vi "Initialize Movement Task.vi"(0 "NI Force Task in":refnum<class "NI Force Task.lvclass">, 1 "Pot Calibration Cluster":cluster{"Left":dbl, "Right":dbl}, 2 "TDMS File":refnum<k34>, 3 "EMG info":cluster{"Collect EMG?":bool, "EMG Rate":u16}, 4 "DAQ  Channels In":T1={"Force Transducer: Left"="Dev1/ai6", "Force Transducer: Right "="Dev1/ai8", "EMG: Left"="", "EMG: Right"="", "Potentiometer: Left"="", "Potentiometer: Right"=""}, 5 "error in (no error)":errorcluster, 7 "Task Info In":T2={"Number of Trials"=1, "Sampling Rate (Hz)"=200, "Trial Duration (s)"=10, "Adjusted MVC (N)"=5.0, "R Phase"=0, "L Phase"=0, "L Pattern"=1, "R Pattern"=1, "Time Between Trials (s)"=5, "Lissajous Speed"=200} {"Lissajous Speed" min=1 max=200; "Time Between Trials (s)" min=1 step=1; "R Pattern" min=1 max=20 step=1; "L Pattern" min=1 max=20 step=1; "L Phase" max=360 step=1; "R Phase" max=360 step=1; "Adjusted MVC (N)" min=1.0 step=1.0; "Trial Duration (s)" min=1 step=1; "Sampling Rate (Hz)" min=1 step=1; "Number of Trials" min=1 step=1}, 9 "Scanning?":bool=TRUE) -> (14 "NI Force Task out":refnum<class "NI Force Task.lvclass">, 19 "error out":errorcluster)   [LabVIEW 2020, in "NI Force Task.lvlib" / "NI Force Task.lvclass"]
uses:
  NI Force Task.lvclass
  C:/Program Files/National Instruments/LabVIEW 2020/vi.lib/ActorFramework/Actor/Actor.lvclass
  Task info df.ctl
  <vilib>/ActorFramework/Message Enqueuer/Message Priority.ctl
  <vilib>/ActorFramework/Actor/Actor.lvclass/Actor.ctl
  <vilib>/ActorFramework/Message Enqueuer/Message Enqueuer.lvclass/Message Enqueuer.ctl
  NI Force Task.lvclass/NI Force Task.ctl
  NI Force Task Messages/Update Template Graph Msg/Update Template Graph Msg.lvclass/Update Template Graph Msg.ctl
  <vilib>/ActorFramework/Message Enqueuer/Init from Existing Queue.vi
  <vilib>/ActorFramework/Message Enqueuer/Enqueue.vi
  NI Force Task Messages/Update Template Graph Msg/Update Template Graph Msg.lvclass
  C:/Program Files/National Instruments/LabVIEW 2020/vi.lib/ActorFramework/Message/Message.lvclass
  <vilib>/ActorFramework/Message Priority Queue/Priority Enqueue.vi
  <vilib>/DAQmx/create/channels.llb/DAQmx Create Channel (AI-Voltage-Basic).vi
  <vilib>/DAQmx/configure/timing.llb/DAQmx Timing (Sample Clock).vi
  <vilib>/ActorFramework/Message Enqueuer/Message Enqueuer.lvclass
  <vilib>/ActorFramework/Actor/Actor.lvclass
panel:
  out "error out 2":errorcluster
  # "Left Arm"
  # "Right Arm"
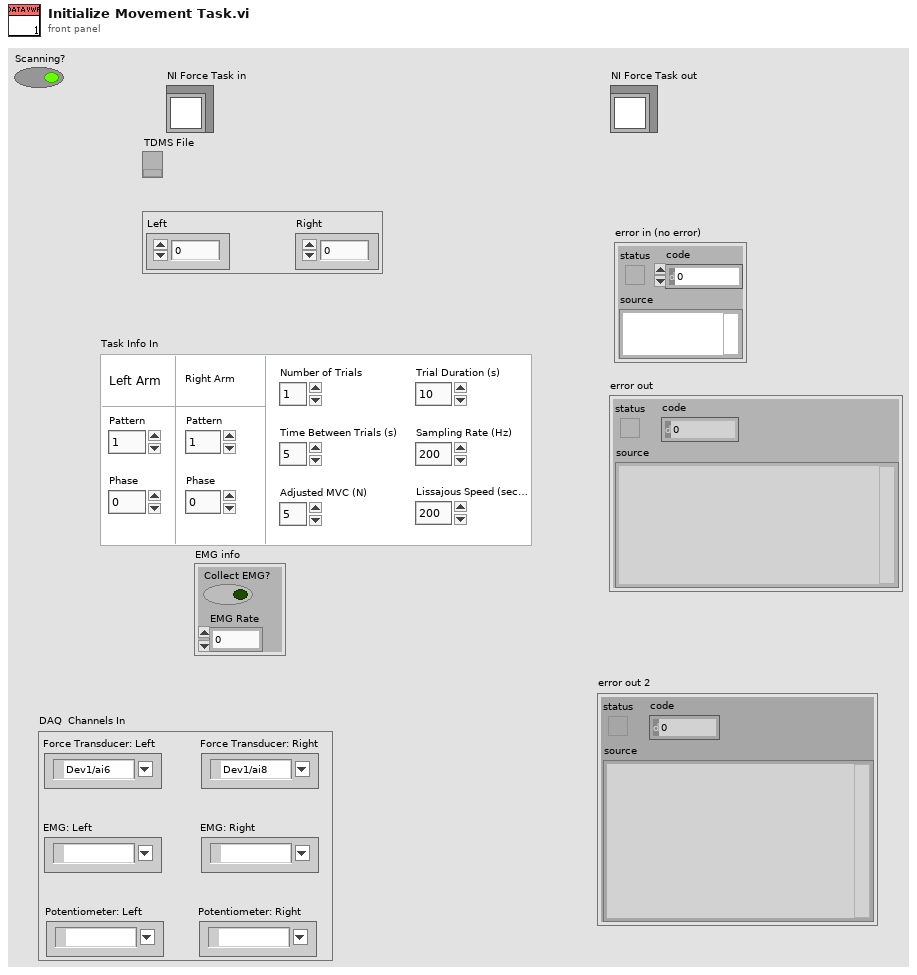
[diagram p1: front panel]
types:
  T1 = cluster{"Force Transducer: Left":tag, "Force Transducer: Right ":tag, "EMG: Left":tag, "EMG: Right":tag, "Potentiometer: Left":tag, "Potentiometer: Right":tag}
  T2 = typedef "Task info df.ctl" = cluster{"Number of Trials":u8, "Sampling Rate (Hz)":u16, "Trial Duration (s)":u8, "Adjusted MVC (N)":dbl, "R Phase":i32, "L Phase":i32, "L Pattern":u8, "R Pattern":u8, "Time Between Trials (s)":u8, "Lissajous Speed":u16}
  T3 = typedef "Actor Framework.lvlib/Message Enqueuer.lvclass/Message Priority.ctl" = enum16{"Low", "Normal", "High"}
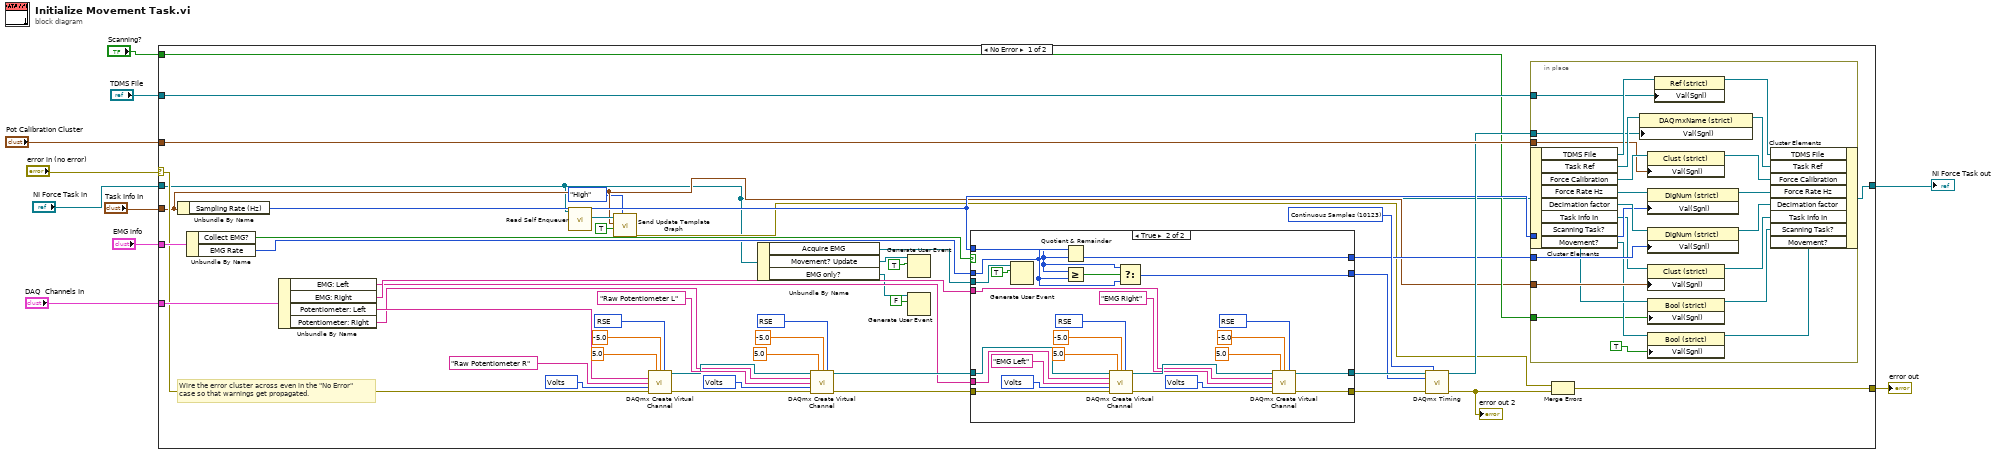
[diagram p0: block diagram]
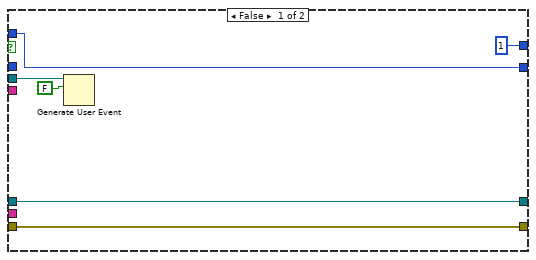
[diagram p2: hidden frame]
diagram:
  n1 = case shown="No Error" "error in (no error)" {
    selector: "error in (no error)" -> [w34 w114]
    tunnel: [w32 w114] -> w9
    tunnel: [w31 w113] -> w7
    tunnel: "NI Force Task in" -> [w13 w113]
    tunnel: "Task Info In" -> [w15 _]
    tunnel: "EMG info" -> [w57 _]
    tunnel: "DAQ  Channels In" -> [w55 _]
    tunnel: "Pot Calibration Cluster" -> [w30 _]
    tunnel: "TDMS File" -> [w28 _]
    tunnel: "Scanning?" -> [w19 _]
    frame No Error {
      w35 = 10123 items=["Finite Samples"=10178, "Continuous Samples"=10123, "Hardware Timed Single Point"=12522] ("sample mode")
      w45 = 10348 items=["Volts"=10348, "From Custom Scale"=10065] ("units")
      w49 = 10083 items=["Default"=-1, "RSE"=10083, "NRSE"=10078, "Differential"=10106, "Pseudodifferential"=12529] ("input terminal configuration")
      w50 = 10348 items=["Volts"=10348, "From Custom Scale"=10065] ("units")
      w54 = 10083 items=["Default"=-1, "RSE"=10083, "NRSE"=10078, "Differential"=10106, "Pseudodifferential"=12529] ("input terminal configuration")
      # "Wire the error cluster across even in the \"No Error\"\ncase so that warnings get propagated."
      n2 = Unbundle By Name(w15) -> ("Sampling Rate (Hz)"=w23:u16)
      n3 = Unbundle By Name(w57) -> ("Collect EMG?"=w56:bool, "EMG Rate"=w36:u16)
      n4 = Unbundle By Name(w55) -> ("EMG: Left"=w25:tag, "EMG: Right"=w26:tag, "Potentiometer: Left"=w42:tag, "Potentiometer: Right"=w41:tag)
      n5 = call <vilib>:"Read Self Enqueuer.vi"("Actor"=w13) -> ("Self Enqueuer"=w16:refnum<class "Message Enqueuer.lvclass">)  [unwired: 10 in]
      n6 = call "Send Update Template Graph.vi"("Priority"=Message_Priority."High", "Update Axes Scale"=TRUE, "Task Info In"=w15, "Message Enqueuer in"=w16) -> ("error out"=w14:errorcluster)  [unwired: 6 in, 1 out]
      n7 = call-poly <vilib>:"DAQmx Create Virtual Channel.vi"("maximum value"=5.0, "minimum value"=-5.0, "input terminal configuration"=w54, "physical channels"=w42, "name to assign"="Raw Potentiometer R", "units"=w50, "error in"=w34) -> ("task out"=w44:refnum<k21>, "error out"=w43:errorcluster)  [unwired: 7 in]
      n8 = Unbundle By Name(w13) -> ("Acquire EMG"=w22:refnum<user-event>, "Movement? Update"=w21:refnum<user-event>, "EMG only?"=w18:refnum<user-event>)
      n9 = call-poly <vilib>:"DAQmx Create Virtual Channel.vi"("task in"=w44, "maximum value"=5.0, "minimum value"=-5.0, "input terminal configuration"=w49, "physical channels"=w41, "name to assign"="Raw Potentiometer L", "units"=w45, "error in"=w43) -> ("task out"=w40:refnum<k21>, "error out"=w39:errorcluster)  [unwired: 6 in]
      n10 = Generate User Event(user event=w21, event data cluster=TRUE ("event data")) -> ()  [unwired: 2 in, 2 out]
      n11 = Generate User Event(user event=w18, event data cluster=FALSE ("event data")) -> ()  [unwired: 2 in, 2 out]
      n12 = case shown="True" w56 {
        tunnel: w40 -> [w63 w78]
        tunnel: [w63 w70] -> w38
        tunnel: [w62 w69] -> w37
        tunnel: w39 -> [w62 w77]
        tunnel: w23 -> [w61 w67]
        tunnel: w36 -> [_ w68]
        tunnel: [w61 w87] -> w27
        tunnel: w26 -> [_ w72]
        tunnel: w25 -> [_ w71]
        tunnel: [u16 1 w66] -> w24
        tunnel: w22 -> [w59 w65]
        frame False {
          n13 = Generate User Event(user event=w59, event data cluster=FALSE ("event data")) -> ()  [unwired: 2 in, 2 out]
        }
        frame True {
          w79 = 10348 items=["Volts"=10348, "From Custom Scale"=10065] ("units")
          w82 = 10083 items=["Default"=-1, "RSE"=10083, "NRSE"=10078, "Differential"=10106, "Pseudodifferential"=12529] ("input terminal configuration")
          w83 = 10348 items=["Volts"=10348, "From Custom Scale"=10065] ("units")
          w86 = 10083 items=["Default"=-1, "RSE"=10083, "NRSE"=10078, "Differential"=10106, "Pseudodifferential"=12529] ("input terminal configuration")
          n14 = Generate User Event(user event=w65, event data cluster=TRUE ("event data")) -> ()  [unwired: 2 in, 2 out]
          n15 = Greater Or Equal?(x=w67, y=w68) -> (x >= y?=w88:bool)
          n16 = Quotient & Remainder(x=w68, y=w67) -> (floor(x/y)=w66:u16)  [unwired: 1 out]
          n17 = call-poly <vilib>:"DAQmx Create Virtual Channel.vi"("task in"=w78, "maximum value"=5.0, "minimum value"=-5.0, "input terminal configuration"=w86, "physical channels"=w71, "name to assign"="EMG Left", "units"=w83, "error in"=w77) -> ("task out"=w76:refnum<k21>, "error out"=w75:errorcluster)  [unwired: 6 in]
          n18 = Select(t=w67, s=w88, f=w68) -> (s? t:f=w87:u16)
          n19 = call-poly <vilib>:"DAQmx Create Virtual Channel.vi"("task in"=w76, "maximum value"=5.0, "minimum value"=-5.0, "input terminal configuration"=w82, "physical channels"=w72, "name to assign"="EMG Right", "units"=w79, "error in"=w75) -> ("task out"=w70:refnum<k21>, "error out"=w69:errorcluster)  [unwired: 6 in]
        }
      }
      n20 = call-poly <vilib>:"DAQmx Timing.vi"("task/channels in"=w38, "sample mode"=w35, "rate"=w27, "error in"=w37) -> ("task out"=w29:refnum<k21>, "error out"=w33:errorcluster)  [unwired: 10 in]
      "error out 2" <- w33
      n21 = in-place {
        in-place-border: w30 -> [w104]
        in-place-border: w29 -> [w110]
        in-place-border: w28 -> [w109]
        in-place-border: w24 -> [w99]
        in-place-border: w23 -> [w98]
        in-place-border: w15 -> [w95]
        in-place-border: w19 -> [w89]
        n22 = in-place-cluster #1(w13) -> ("TDMS File"=w112:refnum<vi>, "Task Ref"=w111:refnum<vi>, "Force Calibration"=w106:refnum<vi>, "Force Rate Hz"=w103:refnum<vi>, "Decimation factor"=w101:refnum<vi>, "Task Info In"=w97:refnum<vi>, "Scanning Task?"=w94:refnum<vi>, "Movement?"=w92:refnum<vi>)
        n23 = property class="DAQmxName (strict)"(reference=w111, "Val(Sgnl)"=w110) -> (reference out=w107:refnum<vi>)  [unwired: 1 in, 1 out]
        n24 = property class="Clust (strict)"(reference=w106, "Val(Sgnl)"=w104) -> (reference out=w105:refnum<vi>)  [unwired: 1 in, 1 out]
        n25 = property class="DigNum (strict)"(reference=w103, "Val(Sgnl)"=w98) -> (reference out=w102:refnum<vi>)  [unwired: 1 in, 1 out]
        n26 = property class="DigNum (strict)"(reference=w101, "Val(Sgnl)"=w99) -> (reference out=w100:refnum<vi>)  [unwired: 1 in, 1 out]
        n27 = property class="Clust (strict)"(reference=w97, "Val(Sgnl)"=w95) -> (reference out=w96:refnum<vi>)  [unwired: 1 in, 1 out]
        n28 = property class="Bool (strict)"(reference=w94, "Val(Sgnl)"=w89) -> (reference out=w93:refnum<vi>)  [unwired: 1 in, 1 out]
        n29 = property class="Bool (strict)"(reference=w92, "Val(Sgnl)"=TRUE ("Value (Signaling)")) -> (reference out=w91:refnum<vi>)  [unwired: 1 in, 1 out]
        n30 = property class="Ref (strict)"(reference=w112, "Val(Sgnl)"=w109) -> (reference out=w108:refnum<vi>)  [unwired: 1 in, 1 out]
        n31 = in-place-cluster #1("TDMS File"=w108, "Task Ref"=w107, "Force Calibration"=w105, "Force Rate Hz"=w102, "Decimation factor"=w100, "Task Info In"=w96, "Scanning Task?"=w93, "Movement?"=w91) -> (w31:refnum<class "NI Force Task.lvclass">)
      }
      n32 = Merge Errors(w14, w33) -> (w32:errorcluster)
    }
    frame Error {
    }
  }
  "error out" <- w9
  "NI Force Task out" <- w7
